vi "Msg.vi"(7 "jettl in":refnum<class "jettl.lvclass">, 11 "Last Ack Creator Msg Strategy in":refnum<class "Last Ack Creator Msg Strategy.lvclass">) -> (5 "jettl out":refnum<class "jettl.lvclass">)   [LabVIEW 2021, in "jettl.lvlib" / "Last Ack Creator Msg Strategy.lvlib" / "Last Ack Creator Msg Strategy.lvclass"]
uses:
  Last Ack Creator Msg Strategy.lvclass
  Last Ack Creator Msg Strategy.lvclass/Last Ack Creator Msg Strategy.ctl
  Last Ack Creator/Last Ack Creator.lvclass
  jettl/jettl.lvclass
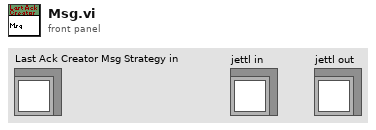
[diagram p1: front panel]
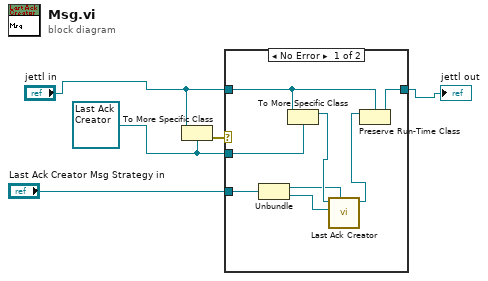
[diagram p0: block diagram]
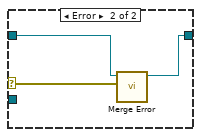
[diagram p2: hidden frame]
diagram:
  w1 = refnum<class "Last Ack Creator.lvclass"> refnum ("jettl.lvlib:jettl Msg Last Ack Creator Queue.lvlib:jettl Msg Last Ack Creator Queue.lvclass")
  n1 = To More Specific Class(target class=w1, reference="jettl in") -> (error out=w5:errorcluster)  [unwired: 1 in, 1 out]
  n2 = case shown="No Error" w5 {
    selector: w5 -> [_ w16]
    tunnel: [w11 w14] -> w3
    tunnel: "jettl in" -> [w12 w15]
    tunnel: w1 -> [w13 _]
    tunnel: "Last Ack Creator Msg Strategy in" -> [w10 _]
    frame No Error {
      n3 = Unbundle "Unbundle"(w10) -> (w6:refnum<class "Sender.lvclass">, w7:refnum<class "jettl.lvclass">)
      n4 = To More Specific Class(target class=w13, reference=w12) -> (specific class reference=w9:refnum<class "Last Ack Creator.lvclass">)  [unwired: 1 in, 1 out]
      n5 = call-dynamic "Last Ack Creator.vi"("Sender"=w6, "jettl"=w7, "Last Ack Creator in"=w9) -> ("Last Ack Creator out"=w8:refnum<class "Last Ack Creator.lvclass">)  [unwired: 8 in]
      n6 = Preserve Run-Time Class(object in=w8, 2:w12) -> (object out=w11:refnum<class "jettl.lvclass">)  [unwired: 1 in, 1 out]
    }
    frame Error {
      n7 = call-dynamic "Merge Error.vi"("Error"=w16, "Merge Error in"=w15) -> ("Merge Error out"=w14:refnum<class "jettl.lvclass">)  [unwired: 9 in]
    }
  }
  "jettl out" <- w3
